vi "Lookup Vacuum Channel.vi"(7 "error in (no error)":errorcluster, 9 "Channel Name":string, 10 "Gantry Class in":refnum<class "Gantry.lvclass">) -> (0 "error out":errorcluster, 2 "Channel Number":i32, 3 "Gantry Class out":refnum<class "Gantry.lvclass">)   [LabVIEW 2023, in "Gantry.lvclass"]
uses:
  Gantry.lvclass
  FlexWorktable/FlexWorktable.lvclass
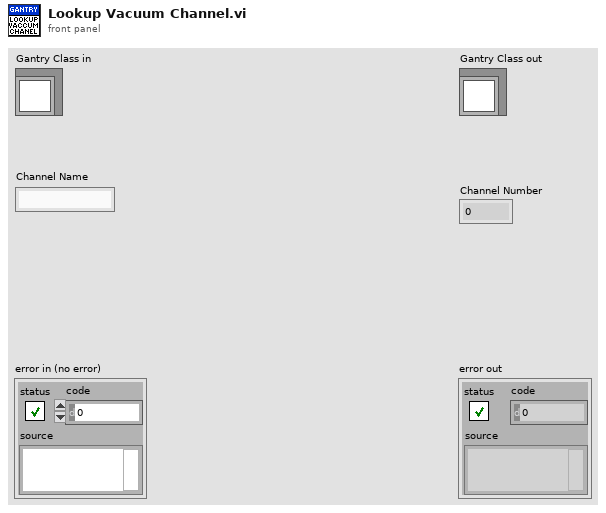
[diagram p1: front panel]
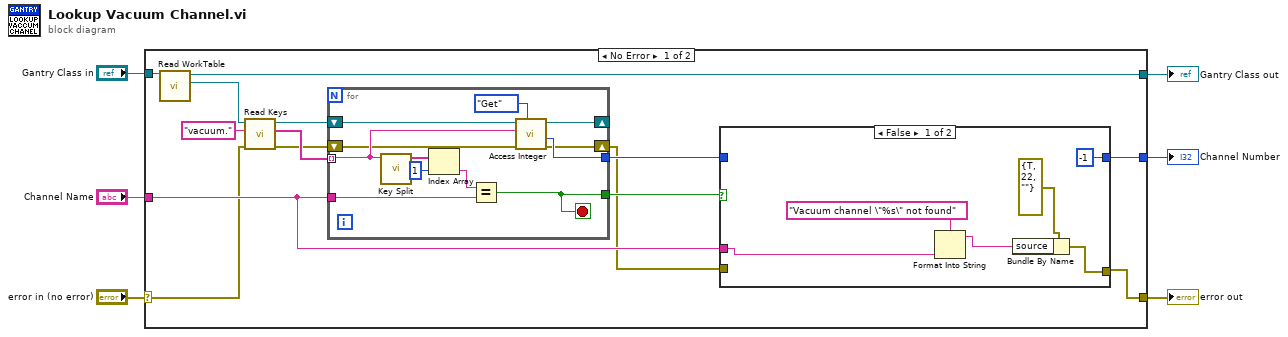
[diagram p0: block diagram]
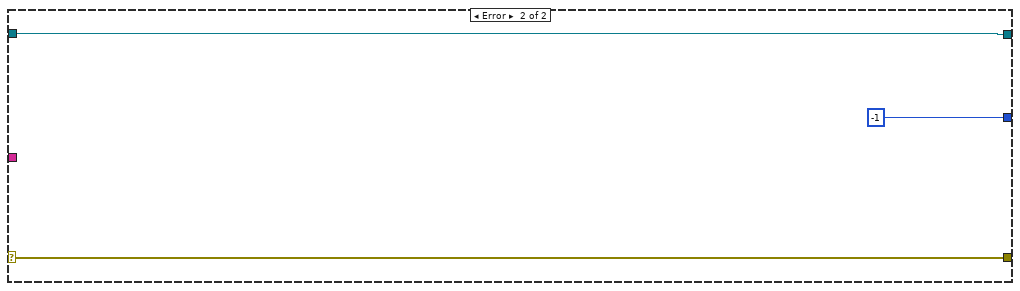
[diagram p3: hidden frame]
diagram:
  n1 = case shown="No Error" "error in (no error)" {
    selector: "error in (no error)" -> [w12 w43]
    tunnel: [w17 w43] -> w5
    tunnel: [w19 w42] -> w3
    tunnel: "Gantry Class in" -> [w20 w42]
    tunnel: "Channel Name" -> [w14 _]
    tunnel: [w15 i8 -1 ("Channel Number")] -> w1
    frame No Error {
      n2 = call-dynamic "Read WorkTable.vi"("Gantry Class in"=w20) -> ("Worktable"=w13:refnum<class "FlexWorktable.lvclass">, "Gantry Class out"=w19:refnum<class "Gantry.lvclass">)  [unwired: 8 in, 1 out]
      n3 = call-dynamic "Read Keys.vi"("error in (no error)"=w12, "Selector"="vacuum.", "FlexWorktable in"=w13) -> ("error out"=w8:errorcluster, "Keys"=w10:string[], "FlexWorktable out"=w9:refnum<class "FlexWorktable.lvclass">)  [unwired: 6 in]
      n4 = for {
        tunnel: w10 -> [w34] mode=indexing
        tunnel: w14 -> [w40]
        tunnel: [w39] -> w18
        tunnel: [w32] -> w16
        shift-right: [w31] -> _
        shift-left: w9 -> [w35]
        shift-right: [w29] -> w7
        shift-left: w8 -> [w30]
        stop <- w39 stop-if-true
        n5 = call "Key Split.vi"("Key"=w34) -> ("Key Elements"=w38:string[])  [unwired: 10 in]
        n6 = Index Array(array=w38, index=1) -> (element=w36:string)
        n7 = Equal?(x=w36, y=w40) -> (x = y?=w39:bool)
        n8 = call-dynamic "Access Integer.vi"("Get/Set"=enum16{"Get", "Set"}."Get", "error in (no error)"=w30, "Key"=w34, "FlexWorktable in"=w35) -> ("error out"=w29:errorcluster, "Value out"=w32:i32, "FlexWorktable out"=w31:refnum<class "FlexWorktable.lvclass">)  [unwired: 5 in]
      }
      n9 = case shown="False" w18 {
        tunnel: w7 -> [_ w28]
        tunnel: [w25 w28] -> w17
        tunnel: w16 -> [_ w27]
        tunnel: [-1 ("Value out") w27] -> w15
        tunnel: w14 -> [w23 _]
        frame False {
          n10 = Format Into String(format string="Vacuum channel \"%s\" not found", w23) -> (resulting string=w22:string)  [unwired: 2 in, 1 out]
          n11 = Bundle By Name(cluster=errorcluster {"status"=TRUE, "code"=22, "source"=""} ("error constant"), "source"=w22) -> (w25:errorcluster)
        }
        frame True {
        }
      }
    }
    frame Error {
    }
  }
  "error out" <- w5
  "Gantry Class out" <- w3
  "Channel Number" <- w1
